vi "Loop.vi"(10 "Queue":refnum<queue>) -> ()   [LabVIEW 2021]
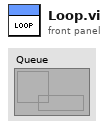
[diagram p1: front panel]
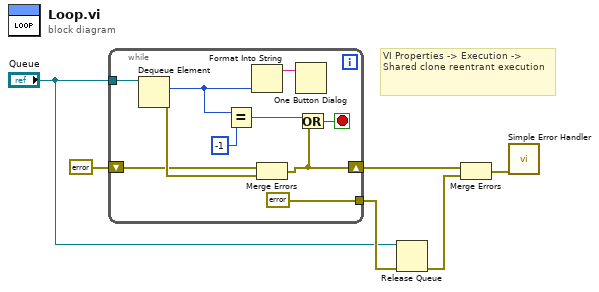
[diagram p0: block diagram]
diagram:
  # "VI Properties -> Execution -> Shared clone reentrant execution"
  n1 = while {
    tunnel: "Queue" -> [w10]
    shift-right: [w7] -> w5
    shift-left: errorcluster {"status"=FALSE, "code"=0, "source"=""} ("error IO") -> [w9]
    tunnel: [errorcluster {"status"=FALSE, "code"=0, "source"=""} ("error in (no error)")] -> w2
    stop <- w8 stop-if-true
    n2 = Dequeue Element(queue=w10) -> (element=w12:i32, error out=w14:errorcluster)  [unwired: 2 in, 2 out]
    n3 = Equal?(x=w12, y=-1) -> (x = y?=w16:bool)
    n4 = Format Into String(w12) -> (resulting string=w13:string)  [unwired: 3 in, 1 out]
    n5 = Merge Errors(w9, w14) -> (w7:errorcluster)
    n6 = One Button Dialog(message=w13) -> ()  [unwired: 1 in, 1 out]
    n7 = Or(x=w16, y=w7) -> (x .or. y?=w8:bool)
  }
  n8 = Release Queue(queue="Queue", error in (no error)=w2) -> (error out=w3:errorcluster)  [unwired: 1 in, 2 out]
  n9 = Merge Errors(w5, w3) -> (w4:errorcluster)
  n10 = call <vilib>:"Simple Error Handler.vi"("error in (no error)"=w4) -> ()  [unwired: 4 in, 5 out]
